vi "get_number_of_pixels.vi"(8 "error in (no error)":errorcluster, 11 "Image in":refnum<class "Image.lvclass">) -> (0 "error out":errorcluster, 2 "number of pixels":i32, 3 "Image out":refnum<class "Image.lvclass">)   [LabVIEW 2010, in "Image.lvclass"]
uses:
  Image.lvclass
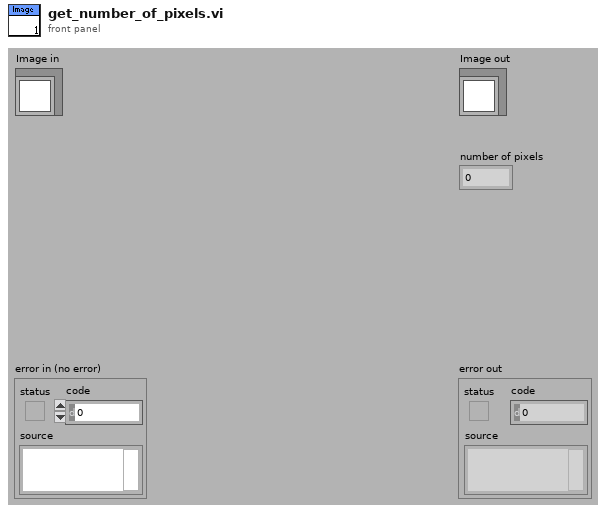
[diagram p1: front panel]
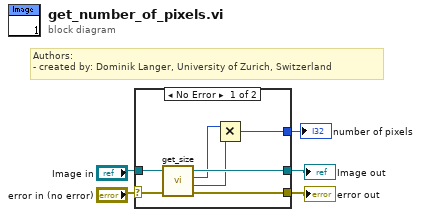
[diagram p0: block diagram]
diagram:
  # "Authors: \n- created by: Dominik Langer, University of Zurich, Switzerland"
  n1 = case shown="No Error" "error in (no error)" {
    selector: "error in (no error)" -> [w10 w14]
    tunnel: [w9 w14] -> w4
    tunnel: [w11 w13] -> w2
    tunnel: "Image in" -> [w12 w13]
    tunnel: [w6 _] -> w1
    frame No Error {
      n2 = call-dynamic "get_size.vi"("error in (no error)"=w10, "Image in"=w12) -> ("error out"=w9:errorcluster, "y resolution"=w7:i32, "x resolution"=w8:i32, "Image out"=w11:refnum<class "Image.lvclass">)  [unwired: 6 out]
      n3 = Multiply(x=w8, y=w7) -> (x*y=w6:i32)
    }
    frame Error {
    }
  }
  "error out" <- w4
  "Image out" <- w2
  "number of pixels" <- w1
